vi "HH_FileToImage_1.vi"(0 "Data In":u32[](array[numeric]), 1 "Reset":bool, 5 "Data Count":i32, 11 "Trace Bins":i32) -> (4 "Histograms":i32[][](array[numeric]), 6 "Total Photon Count":u64[](array[numeric]), 8 "Trigger Times":u64[](array[numeric]), 13 "Total Oveflow Count":u64, 14 "Num Records Total":i64, 15 "Traces":i32[][](array[numeric]))   [LabVIEW 2009]
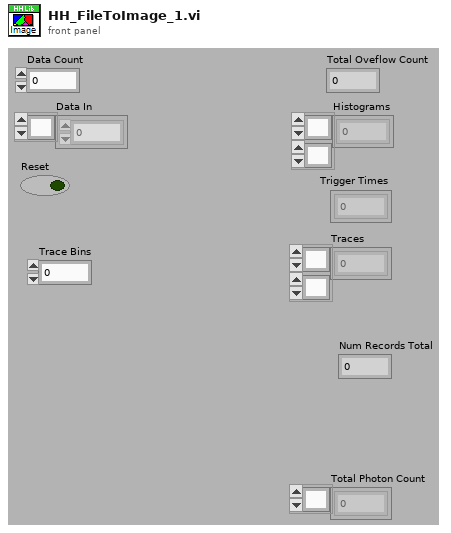
[diagram p1: front panel]
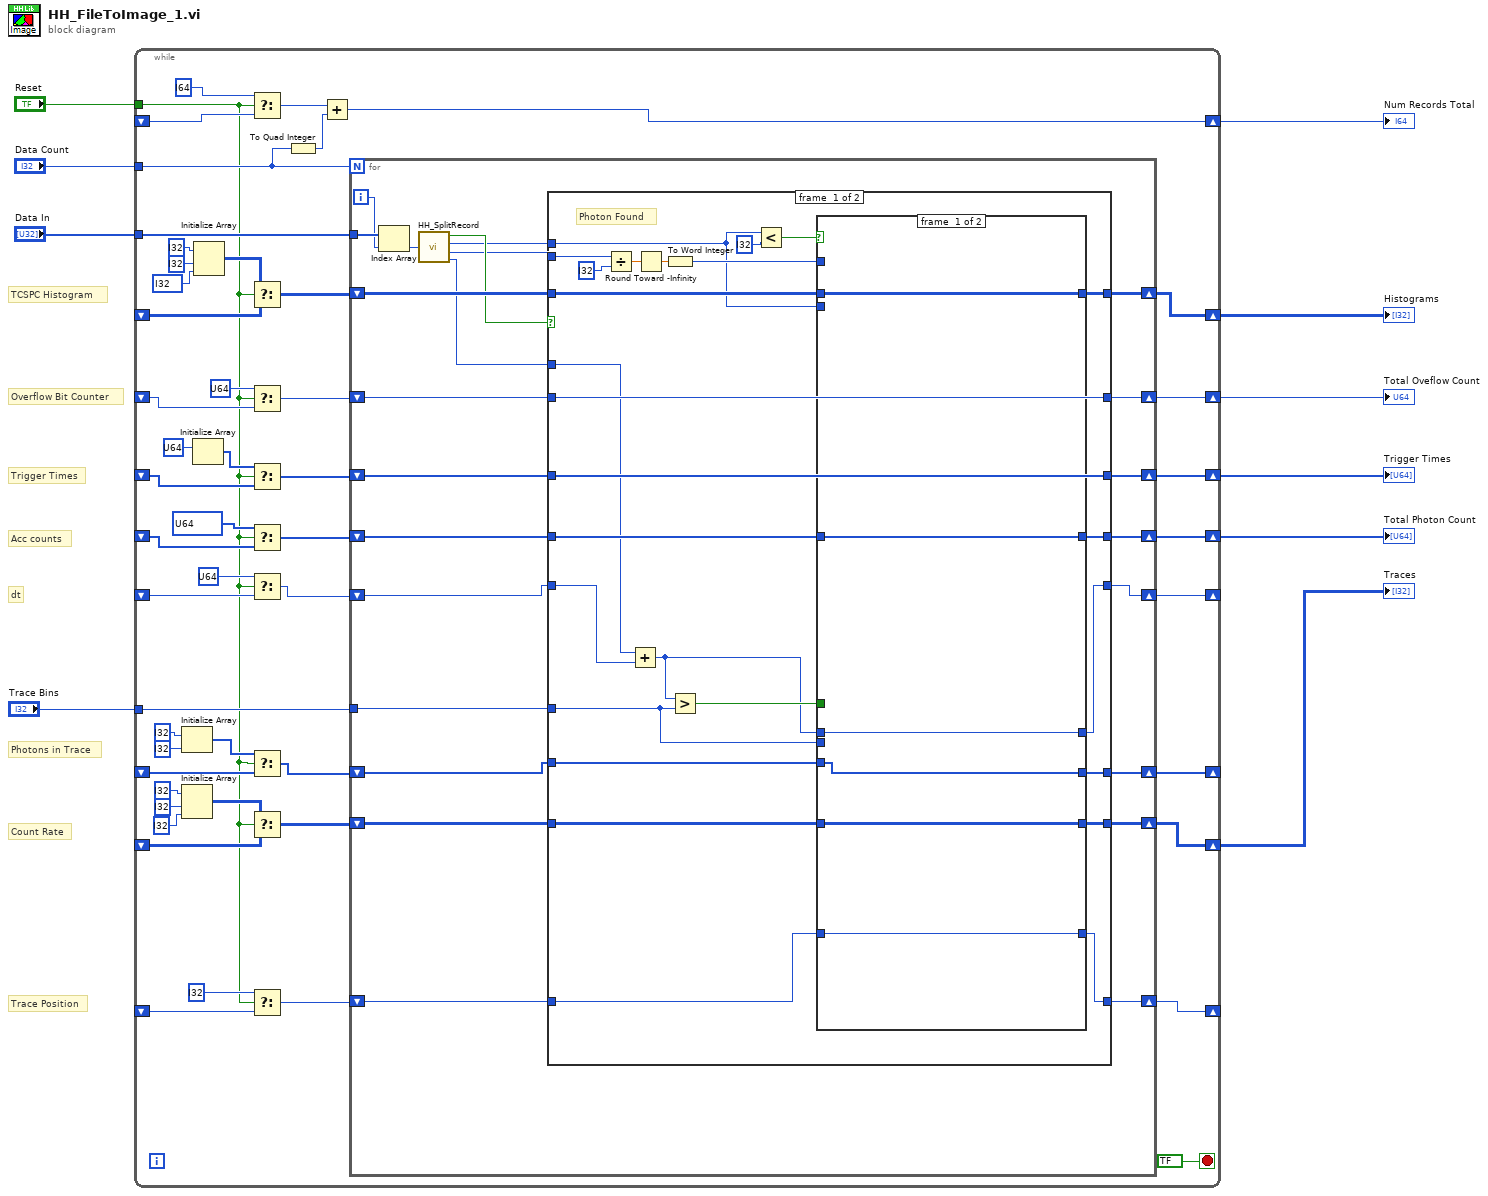
[diagram p0: block diagram]
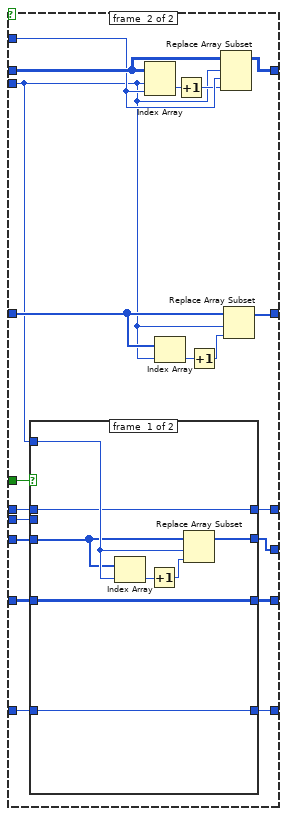
[diagram p2: hidden frame]
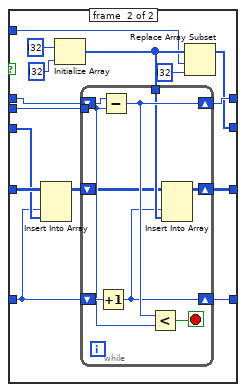
[diagram p3: hidden frame]
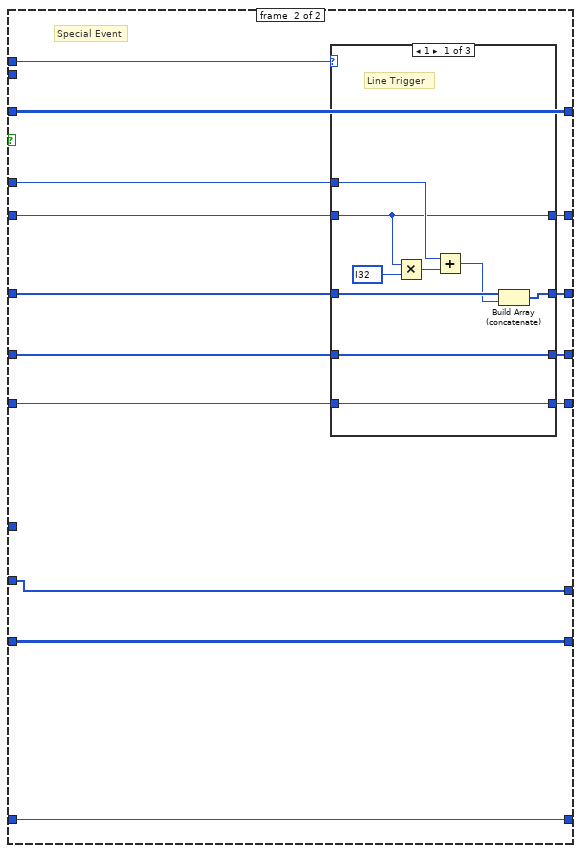
[diagram p4: hidden frame]
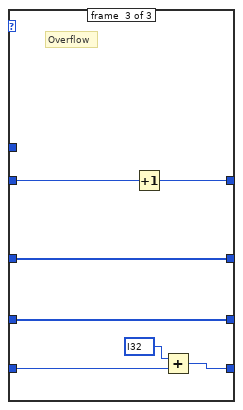
[diagram p6: hidden frame]
diagram:
  # "Photons in Trace"
  # "dt"
  # "Trace Position"
  # "Acc counts"
  # "Count Rate"
  # "Trigger Times"
  # "TCSPC Histogram"
  # "Overflow Bit Counter"
  n1 = while {
    tunnel: "Data In" -> [w59]
    shift-right: [w60] -> w10
    shift-left: _ -> [w55]
    tunnel: "Reset" -> [w12]
    shift-right: [w52] -> w3
    shift-left: _ -> [w51]
    shift-right: [w47] -> w7
    shift-left: _ -> [w46]
    shift-right: [w42] -> w6
    shift-left: _ -> [w41]
    tunnel: "Trace Bins" -> [w40]
    shift-right: [w37] -> _
    shift-left: _ -> [w36]
    tunnel: "Data Count" -> [w24]
    shift-right: [w32] -> w4
    shift-left: _ -> [w34]
    shift-right: [w26] -> w2
    shift-left: _ -> [w25]
    shift-right: [w20] -> _
    shift-left: _ -> [w19]
    shift-right: [w14] -> _
    shift-left: _ -> [w13]
    stop <- bool ? stop-if-true
    n2 = Initialize Array(i32 ? ("element"), i32 ? ("dimension size")) -> (w17:i32[])
    n3 = Initialize Array(i32 ? ("element"), i32 ? ("dimension size"), i32 ?) -> (w44:i32[][])
    n4 = Initialize Array(u64 ? ("element")) -> (w49:u64[])  [unwired: 1 out]
    n5 = Initialize Array(i32 ? ("element"), i32 ? ("dimension size"), i32 ? ("dimension size")) -> (w56:i32[][])
    n6 = Select(t=i64 ? ("Data Count 2"), s=w12, f=w34) -> (s? t:f=w33:i64)
    n7 = Select(t=w56, s=w12, f=w55) -> (s? t:f=w57:i32[][])
    n8 = Select(t=u64 ?, s=w12, f=w51) -> (s? t:f=w53:u64)
    n9 = Select(t=w49, s=w12, f=w46) -> (s? t:f=w48:u64[])
    n10 = Select(t=u64[] ? ("initialized array"), s=w12, f=w25) -> (s? t:f=w27:u64[])
    n11 = Select(t=u64 ?, s=w12, f=w19) -> (s? t:f=w21:u64)
    n12 = Select(t=w17, s=w12, f=w13) -> (s? t:f=w15:i32[])
    n13 = Select(t=w44, s=w12, f=w41) -> (s? t:f=w43:i32[][])
    n14 = Select(t=i32 ?, s=w12, f=w36) -> (s? t:f=w38:i32)
    n15 = To Quad Integer(1:w24) -> (0:w23:i64)
    n16 = Add(x=w33, y=w23) -> (x+y=w32:i64)
    n17 = for {
      N: w24 -> [_]
      tunnel: w59 -> [w79]
      shift-right: [w84] -> w60
      shift-left: w57 -> [w85]
      shift-right: [w82] -> w52
      shift-left: w53 -> [w83]
      shift-right: [w80] -> w47
      shift-left: w48 -> [w81]
      shift-right: [w62] -> w42
      shift-left: w43 -> [w67]
      tunnel: w40 -> [w66]
      shift-right: [w63] -> w37
      shift-left: w38 -> [w68]
      shift-right: [w76] -> w26
      shift-left: w27 -> [w77]
      shift-right: [w64] -> w14
      shift-left: w15 -> [w65]
      shift-right: [w71] -> w20
      shift-left: w21 -> [w70]
      i -> [w78]
      n18 = Index Array(array=w79, index=w78) -> (element=w75:u32)
      n19 = call "HH_SplitRecord.vi"("Record in"=w75) -> ("Special"=w74:bool, "channel"=w73:i32, "time"=w72:i32, "nsync"=w69:u16)
      n20 = case shown="True" w74 {
        tunnel: w85 -> [w111 w181]
        tunnel: w73 -> [w94 w176]
        tunnel: [w110 w181] -> w84
        tunnel: w72 -> [w103 _]
        tunnel: w83 -> [w109 w183]
        tunnel: [w109 w182] -> w82
        tunnel: w81 -> [w108 w180]
        tunnel: [w108 w179] -> w80
        tunnel: w69 -> [w99 w170]
        tunnel: w77 -> [w105 w178]
        tunnel: [w104 w177] -> w76
        tunnel: w70 -> [w89 w175]
        tunnel: [w90 w174] -> w71
        tunnel: w67 -> [w97 w172]
        tunnel: w68 -> [w98 w173]
        tunnel: w66 -> [w87 _]
        tunnel: w65 -> [w96 w171]
        tunnel: [w91 w171] -> w64
        tunnel: [w93 w173] -> w63
        tunnel: [w92 w172] -> w62
        frame #0 {
          # "Photon Found"
          n21 = Divide(x=w103, y=i32 ?) -> (x/y=w102:dbl)
          n22 = Add(x=w99, y=w89) -> (x+y=w88:u64)
          n23 = Round Toward -Infinity(1:w102) -> (0:w86:dbl)
          n24 = To Word Integer(number=w86) -> (16bit integer=w100:i16)
          n25 = Greater?(x=w88, y=w87) -> (0:w95:bool)
          n26 = Less?(x=w94, y=i32 ?) -> (x < y?=w107:bool)
          n27 = case shown="True" w107 {
            tunnel: w111 -> [w117 w137]
            tunnel: [w117 w136] -> w110
            tunnel: w100 -> [_ w135]
            tunnel: w94 -> [_ w121]
            tunnel: w105 -> [w116 w130]
            tunnel: [w116 w129] -> w104
            tunnel: w98 -> [w115 w128]
            tunnel: w97 -> [w114 w127]
            tunnel: w96 -> [w113 w126]
            tunnel: w88 -> [w112 w120]
            tunnel: w95 -> [_ w125]
            tunnel: [w115 w124] -> w93
            tunnel: [w114 w123] -> w92
            tunnel: [w113 w122] -> w91
            tunnel: [w112 w119] -> w90
            tunnel: w87 -> [_ w118]
            frame #0 {
            }
            frame #1 {
              n28 = case shown="True" w125 {
                tunnel: w127 -> [w144 w160]
                tunnel: w128 -> [w145 w146]
                tunnel: [w144 w151] -> w123
                tunnel: [w145 w153] -> w124
                tunnel: w121 -> [w141 w147]
                tunnel: w126 -> [w139 w155]
                tunnel: [w140 w150] -> w122
                tunnel: w120 -> [w138 w156]
                tunnel: [w138 w157] -> w119
                tunnel: w118 -> [_ w154]
                frame #0 {
                  n29 = Index Array(array=w139, index=w141) -> (element=w142:i32)
                  n30 = Increment(x=w142) -> (x+1=w143:i32)
                  n31 = Replace Array Subset(array=w139, new element=w143, index=w141) -> (w140:i32[])
                }
                frame #1 {
                  n32 = Insert Into Array(array=w160, index (col)=w146, new element=w155) -> (w152:i32[][])  [unwired: 1 in]
                  n33 = Initialize Array(i32 ?, i32 ?) -> (w149:i32[])
                  n34 = while {
                    tunnel: w154 -> [w165]
                    tunnel: w149 -> [w164]
                    shift-right: [w162] -> w151
                    shift-left: w152 -> [w163]
                    shift-right: [w161] -> w153
                    shift-left: w146 -> [w168]
                    shift-right: [w166] -> w157
                    shift-left: w156 -> [w169]
                    stop <- w167 stop-if-true
                    n35 = Increment(x=w168) -> (x+1=w161:i32)
                    n36 = Subtract(x=w169, y=w165) -> (x-y=w166:u64)
                    n37 = Less?(x=w166, y=w165) -> (x < y?=w167:bool)
                    n38 = Insert Into Array(array=w163, index (col)=w161, new element=w164) -> (w162:i32[][])  [unwired: 1 in]
                  }
                  n39 = Replace Array Subset(array=w149, new element=i32 ?, index=w147) -> (w150:i32[])
                }
              }
              n40 = Index Array(array=w137, index (row)=w121, index (col)=w135) -> (element=w134:i32)
              n41 = Index Array(array=w130, index=w121) -> (element=w132:u64)
              n42 = Increment(x=w134) -> (x+1=w133:i32)
              n43 = Increment(x=w132) -> (x+1=w131:u64)
              n44 = Replace Array Subset(array=w137, new element=w133, index (row)=w121, index (col)=w135) -> (w136:i32[][])
              n45 = Replace Array Subset(array=w130, new element=w131, index=w121) -> (w129:u64[])
            }
          }
        }
        frame #1 {
          # "Special Event"
          n46 = case shown="1" w176 {
            tunnel: w183 -> [w185 w196 w202]
            tunnel: [w185 w196 w201] -> w182
            tunnel: w180 -> [w192 w195 w203]
            tunnel: [w191 w195 w203] -> w179
            tunnel: w178 -> [w190 w194 w200]
            tunnel: [w190 w194 w200] -> w177
            tunnel: w175 -> [w188 w193 w199]
            tunnel: [w188 w193 w197] -> w174
            tunnel: w170 -> [w187 _ _]
            frame #0 {
              # "Line Trigger"
              n47 = Multiply(x=w185, y=i32 ?) -> (x*y=w186:u64)
              n48 = Add(x=w187, y=w186) -> (x+y=w189:u64)
              n49 = Build Array (concatenate)(w192, w189) -> (w191:u64[])
            }
            frame #1 {
            }
            frame #2 {
              # "Overflow"
              n50 = Increment(x=w202) -> (x+1=w201:u64)
              n51 = Add(x=i32 ?, y=w199) -> (x+y=w197:u64)
            }
          }
        }
      }
    }
  }
  "Histograms" <- w10
  "Trigger Times" <- w7
  "Traces" <- w6
  "Num Records Total" <- w4
  "Total Oveflow Count" <- w3
  "Total Photon Count" <- w2
